vi "Pre Launch Init.vi"(11 "Base UI Component in":refnum<class "Base UI Component.lvclass">) -> (0 "error out":errorcluster, 3 "Base UI Component out":refnum<class "Base UI Component.lvclass">)   [LabVIEW 2016, in "Assert Display.lvlib" / "Base UI Component.lvlib" / "Base UI Component.lvclass"]
doc: "(<B>Filename</B>: Actor Framework.lvlib:Actor.lvclass:Pre Launch Init.vi)\n\nDefines behavior that occurs after the Launch Nested Actor method is invoked but before the actor's Actor Core method begins running.\n\nBy default, this method does nothing. A descendant class may override it to define behavior."
uses:
  Base UI Component.lvclass
  Base UI Component.lvclass/Base UI Component.ctl
  Base UI Actor/Base UI Actor/Base UI Actor.lvclass
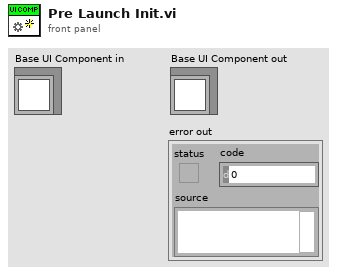
[diagram p1: front panel]
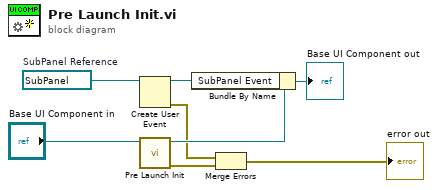
[diagram p0: block diagram]
diagram:
  w5 = refnum<vi> refnum  # SubPanel Reference
  n1 = Create User Event(user event datatype=w5) -> (user event=w3:refnum<user-event>, error out=w1:errorcluster)  [unwired: 1 in]
  n2 = call-parent "Pre Launch Init.vi"("Base UI Actor in"="Base UI Component in") -> ("error out"=w8:errorcluster, "Base UI Actor out"=w7:refnum<class "Base UI Component.lvclass">)  [unwired: 9 in]
  n3 = Bundle By Name(cluster=w7, "SubPanel Event"=w3) -> (→"Base UI Component out":refnum<class "Base UI Component.lvclass">)
  n4 = Merge Errors(w1, w8) -> (→"error out":errorcluster)
